vi "Export Trigger Pulse (Stretched).vi"(2 "FPGA I/O Pin":refnum<k21>="PXI_Trig0", 7 "Input Signal":bool) -> ()   [LabVIEW 2012]
uses:
  <vilib>/rvi/eio/common/nirviEmuTemplateMethod_errors.vi
  <vilib>/eio/EIONode/EIONode.xnode
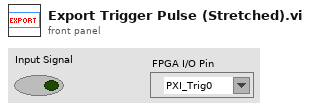
[diagram p1: front panel]
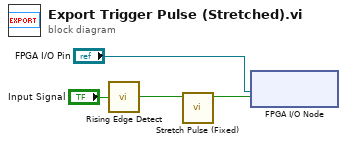
[diagram p0: block diagram]
diagram:
  n1 = call <userlib>:"Rising Edge Detect.vi"("signal"="Input Signal") -> ("edge detected"=w4:bool)  [unwired: 14 in]
  n2 = call <userlib>:"Stretch Pulse (Fixed).vi"("Pulse"=w4) -> ("Stretched Pulse"=w3:bool)  [unwired: 10 in]
  n3 = xnode "FPGA I/O Node"("I/O Item"=w3, "FPGA I/O In"="FPGA I/O Pin") -> ()  [unwired: 1 out]
